vi "Autosize Clear Error All or Specified.vi"(6 "Clear Mode (0: Clear All)":enum16{"Clear All", "Clear Specified"}(ring), 8 "Code to Clear (0)":i32, 10 "Code to Clear [ ]":i32[](array[numeric]), 14 "error in (no error)":errorcluster) -> (3 "error out":errorcluster)   [LabVIEW 2015]
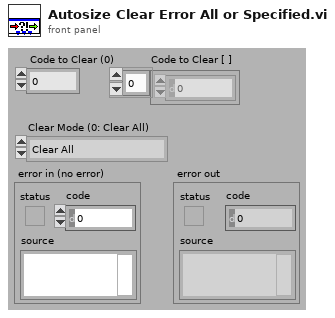
[diagram p1: front panel]
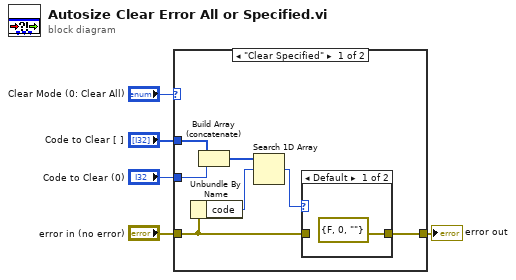
[diagram p0: block diagram]
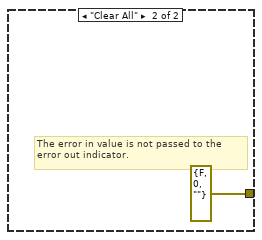
[diagram p3: hidden frame]
diagram:
  n1 = case shown="\"Clear Specified\"" "Clear Mode (0: Clear All)" {
    tunnel: "error in (no error)" -> [w12 _]
    tunnel: [w11 errorcluster {"status"=FALSE, "code"=0, "source"=""} ("error in (no error)")] -> w2
    tunnel: "Code to Clear [ ]" -> [w7 _]
    tunnel: "Code to Clear (0)" -> [w6 _]
    frame "Clear Specified" {
      n2 = Unbundle By Name(w12) -> ("code"=w9:i32)
      n3 = Build Array (concatenate)(w7, w6) -> (w10:i32[])
      n4 = Search 1D Array(1D array=w10, element=w9) -> (index of element=w8:i32)  [unwired: 1 out]
      n5 = case shown="Default" w8 {
        tunnel: w12 -> [_ w14]
        tunnel: [errorcluster {"status"=FALSE, "code"=0, "source"=""} ("error in (no error)") w14] -> w11
        frame Default {
        }
        frame -1 {
        }
      }
    }
    frame "Clear All" {
      # "The error in value is not passed to the\nerror out indicator."
    }
  }
  "error out" <- w2
